vi "Wave2D_Init Data_Start Idx and Length.vi"(10 "Boundary Condition":cluster{"type":T2, "Value":dbl[][]}[](array[cluster]) {"type" items=["Dirichlet", "Neumann"]}, 11 "Domain":T1={"t"={"initial t"=0.0, "final t"=1.0, "# of t-points"=11}, "x"={"start x"=0.0, "end x"=1.0, "# of x-points"=11}, "y"={"start y"=0.0, "end y"=1.0, "# of y-points"=11}}) -> (0 "y length":i32, 1 "y start index":i32, 2 "x length":i32, 3 "x start index":i32)   [LabVIEW 2017, in "NI_PDE.lvlib"]
uses:
  <vilib>/gmath/NI_PDE.lvlib
  <vilib>/gmath/pde.llb/Common/PDE_BC Type.ctl
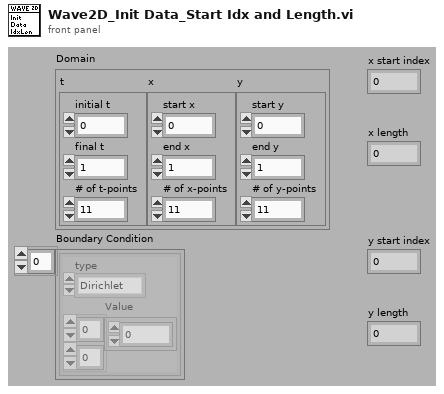
[diagram p1: front panel]
types:
  T1 = cluster{"t":cluster{"initial t":dbl, "final t":dbl, "# of t-points":i32}, "x":cluster{"start x":dbl, "end x":dbl, "# of x-points":i32}, "y":cluster{"start y":dbl, "end y":dbl, "# of y-points":i32}}
  T2 = typedef "NI_PDE.lvlib/PDE_BC Type.ctl" = i32
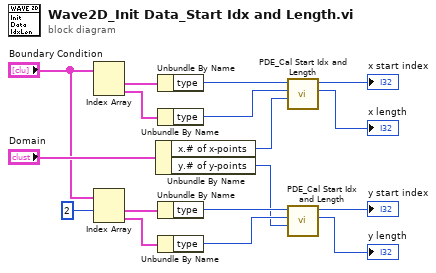
[diagram p0: block diagram]
diagram:
  n1 = Index Array(array="Boundary Condition") -> (element #1=w17:cluster{"type":T2, "Value":dbl[][]}, element #2=w16:cluster{"type":T2, "Value":dbl[][]})  [unwired: 2 in]
  n2 = Index Array(array="Boundary Condition", index #1=2 ("index")) -> (element #1=w13:cluster{"type":T2, "Value":dbl[][]}, element #2=w14:cluster{"type":T2, "Value":dbl[][]})  [unwired: 1 in]
  n3 = Unbundle By Name("Domain") -> ("x.# of x-points"=w6:i32, "y.# of y-points"=w3:i32)
  n4 = Unbundle By Name(w17) -> ("type"=w10:T2)
  n5 = Unbundle By Name(w16) -> ("type"=w9:T2)
  n6 = Unbundle By Name(w13) -> ("type"=w5:T2)
  n7 = Unbundle By Name(w14) -> ("type"=w4:T2)
  n8 = call <vilib>:"PDE_Cal Start Idx and Length.vi"("# of points"=w6, "end type"=w9, "start type"=w10) -> ("length"=→"x length":i32, "start index"=→"x start index":i32)  [unwired: 7 out]
  n9 = call <vilib>:"PDE_Cal Start Idx and Length.vi"("# of points"=w3, "end type"=w4, "start type"=w5) -> ("length"=→"y length":i32, "start index"=→"y start index":i32)  [unwired: 7 out]
